vi "CH_LM App Dispatcher.vi"(3 "Menu occurrence":refnum<k4>, 4 "error in (no error)":errorcluster, 5 "Device disable occurrence":refnum<k4>, 6 "MainGUI?":bool, 7 "Stop Main Occurrence":refnum<k4>) -> (0 "error out":errorcluster)   [LabVIEW 2012, in "CH_LM App.lvlib"]
doc: "This VI is used to dispatch new LabMax PC frontpanels."
uses:
  CH_LM App.lvlib
  CH_LM App FGV Functions.ctl
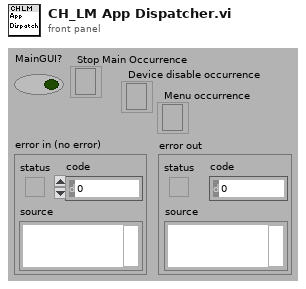
[diagram p1: front panel]
types:
  T1 = typedef "CH_LM App.lvlib/CH_LM App FGV Functions.ctl" = enum16{"create", "get", "set", "remove", "clear", "getBySerial"}
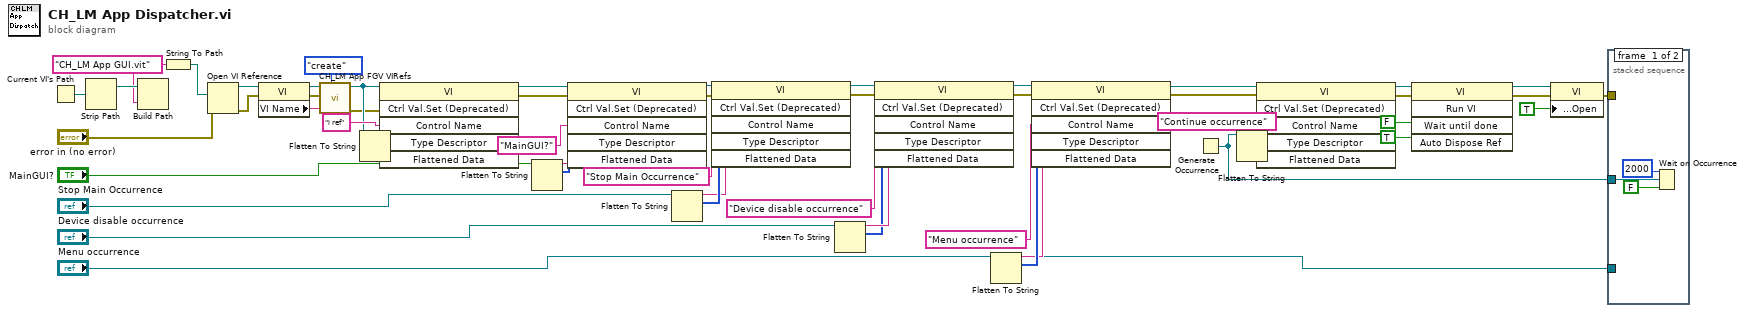
[diagram p0: block diagram]
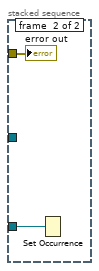
[diagram p2: hidden frame]
diagram:
  w3 = "CH_LM App GUI.vit"
  n1 = Current VI's Path() -> (path=w54:path)
  n2 = Strip Path(path=w54) -> (stripped path=w53:path)  [unwired: 1 out]
  n3 = Build Path(base path=w53, name or relative path=w3) -> ()  [unwired: 1 out]
  n4 = String To Path(string=w3) -> (path=w4:path)
  n5 = Open VI Reference(vi path=w4, error in (no error)="error in (no error)") -> (vi reference=w34:refnum<vi>, error out=w33:errorcluster)  [unwired: 4 out]
  n6 = property class="VI"(reference=w34, error in=w33) -> (reference out=w31:refnum<vi>, error out=w32:errorcluster, "VI Name"=w30:string)
  n7 = call "CH_LM App FGV VIRefs.vi"("Function"=CH_LM_App_FGV_Functions."create", "error in (no error)"=w32, "VI Name"=w30, "VI Ref"=w31) -> ("error out"=w7:errorcluster, "VI Ref"=w9:refnum<vi>)  [unwired: 6 out]
  n8 = Flatten To String(anything=w9) -> (data string=w12:string, type string=w11:i16[])  [unwired: 1 in, 3 out]
  n9 = invoke class="VI" method="Ctrl Val.Set (Deprecated)"(reference=w9, error in=w7, "Control Name"="i ref", "Type Descriptor"=w11, "Flattened Data"=w12) -> (reference out=w8:refnum<vi>, error out=w6:errorcluster)  [unwired: 1 in, 4 out]
  n10 = Flatten To String(anything="MainGUI?") -> (data string=w44:string, type string=w43:i16[])  [unwired: 1 in, 3 out]
  n11 = invoke class="VI" method="Ctrl Val.Set (Deprecated)"(reference=w8, error in=w6, "Control Name"="MainGUI?", "Type Descriptor"=w43, "Flattened Data"=w44) -> (reference out=w38:refnum<vi>, error out=w39:errorcluster)  [unwired: 1 in, 4 out]
  n12 = Flatten To String(anything="Stop Main Occurrence") -> (data string=w40:string, type string=w41:i16[])  [unwired: 1 in, 3 out]
  n13 = invoke class="VI" method="Ctrl Val.Set (Deprecated)"(reference=w38, error in=w39, "Control Name"="Stop Main Occurrence", "Type Descriptor"=w41, "Flattened Data"=w40) -> (reference out=w27:refnum<vi>, error out=w26:errorcluster)  [unwired: 1 in, 4 out]
  n14 = Flatten To String(anything="Device disable occurrence") -> (data string=w29:string, type string=w28:i16[])  [unwired: 1 in, 3 out]
  n15 = invoke class="VI" method="Ctrl Val.Set (Deprecated)"(reference=w27, error in=w26, "Control Name"="Device disable occurrence", "Type Descriptor"=w28, "Flattened Data"=w29) -> (reference out=w23:refnum<vi>, error out=w22:errorcluster)  [unwired: 1 in, 4 out]
  n16 = Flatten To String(anything="Menu occurrence") -> (data string=w17:string, type string=w18:i16[])  [unwired: 1 in, 3 out]
  n17 = invoke class="VI" method="Ctrl Val.Set (Deprecated)"(reference=w23, error in=w22, "Control Name"="Menu occurrence", "Type Descriptor"=w18, "Flattened Data"=w17) -> (reference out=w21:refnum<vi>, error out=w20:errorcluster)  [unwired: 1 in, 4 out]
  n18 = Generate Occurrence() -> (w5:refnum<k4>)
  n19 = Flatten To String(anything=w5) -> (data string=w46:string, type string=w47:i16[])  [unwired: 1 in, 3 out]
  n20 = invoke class="VI" method="Ctrl Val.Set (Deprecated)"(reference=w21, error in=w20, "Control Name"="Continue occurrence", "Type Descriptor"=w47, "Flattened Data"=w46) -> (reference out=w51:refnum<vi>, error out=w49:errorcluster)  [unwired: 1 in, 4 out]
  n21 = invoke class="VI" method="Run VI"(reference=w51, error in=w49, "Wait until done"=FALSE, "Auto Dispose Ref"=TRUE) -> (reference out=w16:refnum<vi>, error out=w15:errorcluster)  [unwired: 1 in, 3 out]
  n22 = property class="VI"(reference=w16, error in=w15, "Front Panel Window:Open"=TRUE) -> (error out=w45:errorcluster)  [unwired: 1 out]
  n23 = stacked-sequence {
    tunnel: w45 -> [_ w59]
    tunnel: "Menu occurrence" -> [_ w58]
    tunnel: w5 -> [w56 _]
    frame #0 {
      n24 = Wait on Occurrence(1:FALSE ("ignore previous (T)"), 2:w56, 3:u32 2000 ("milliseconds to wait")) -> ()  [unwired: 1 out]
    }
    frame #1 {
      n25 = Set Occurrence(w58) -> ()
      "error out" <- w59
    }
  }
